vi "SmartInsert.vi"(8 "error in (no error)":errorcluster, 11 "SelList[]":refnum<vi>[](array[refnum])) -> (0 "error out":errorcluster)   [LabVIEW 2014]
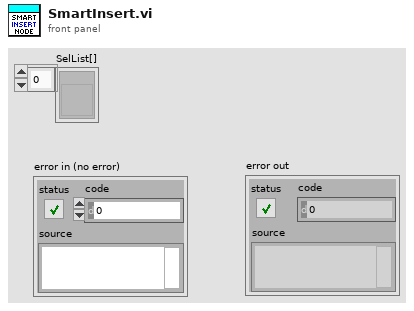
[diagram p1: front panel]
types:
  T1 = cluster{"Source":refnum<vi>, "Sink":refnum<vi>, "Type Variant":variant}
  T2 = cluster{"Position":cluster{"h":i16, "v":i16}, "Flags":i32, "Type":enum32{"LooseEnd", "Endpoint", "Bend", "Junction"}, "Up Joint Index":i16, "Down Joint Index":i16, "Left Joint Index":i16, "Right Joint Index":i16}[]
  T3 = typedef "LVPointTypeDef.ctl" = cluster{"Horizontal":i16, "Vertical":i16}
  T4 = typedef "LVPositionTypeDef.ctl" = cluster{"Left":i32, "Top":i32}
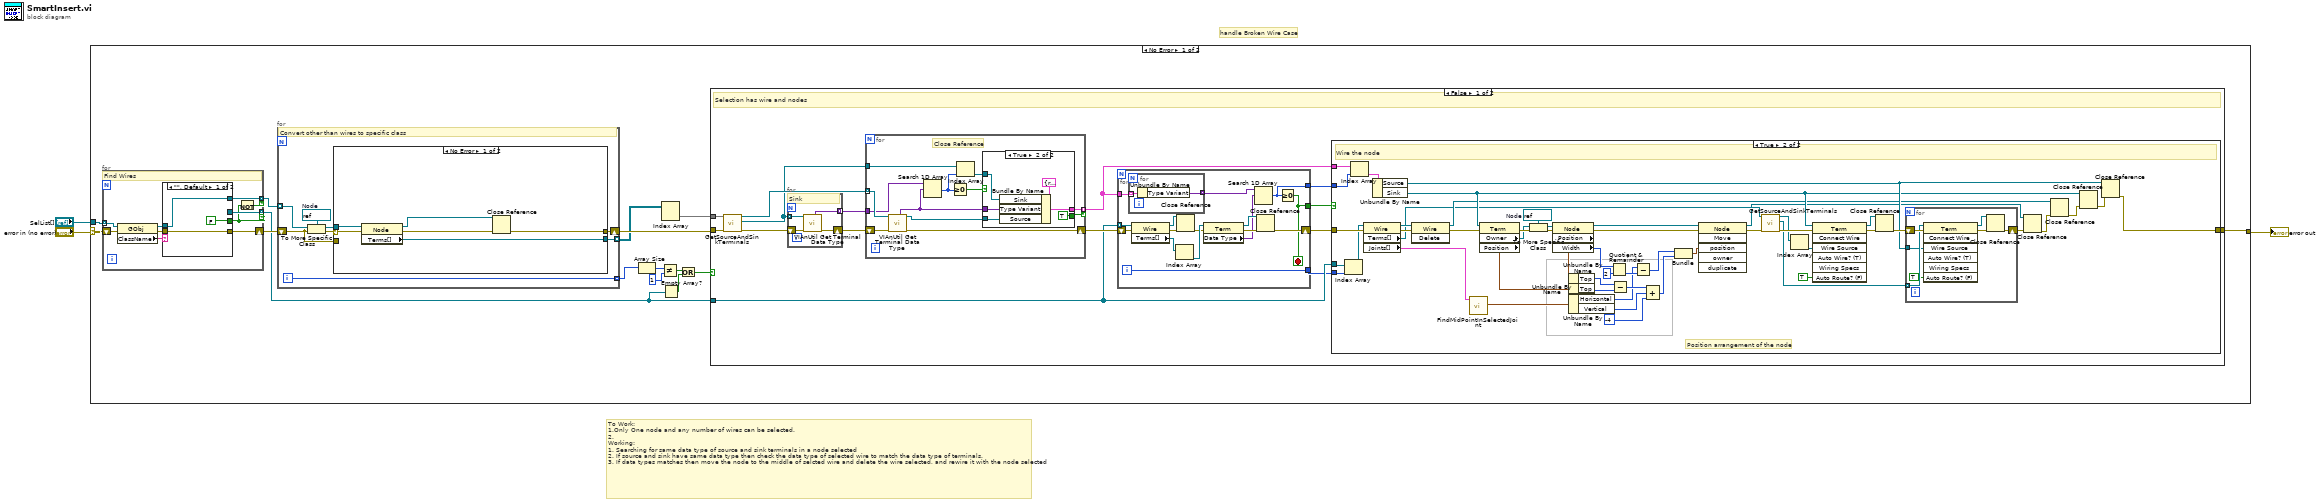
[diagram p0: block diagram]
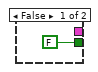
[diagram p3: hidden frame]
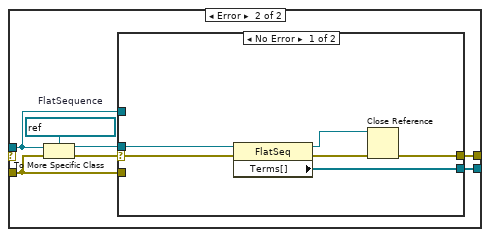
[diagram p5: hidden frame]
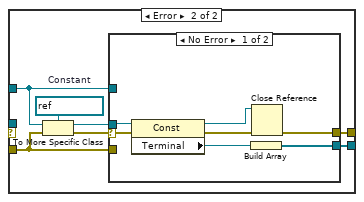
[diagram p6: hidden frame]
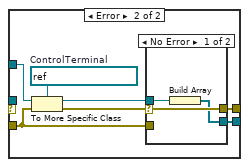
[diagram p7: hidden frame]
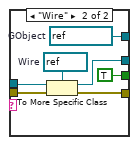
[diagram p9: hidden frame]
diagram:
  # "To Work:\n1.Only One node and any number of wires can be selected.\n2.\nWorking:\n1. Searching for same data type of source and sink terminals in a node selected\n2. If source and sink have same data type then check the data type of selected wire to match the data type of terminals.\n3. If data types matches then move the node to the middle of selcted wire and delete the wire selected, and rewire it with the node selected"
  # "handle Broken Wire Case"
  n1 = case shown="No Error" "error in (no error)" {
    selector: "error in (no error)" -> [w17 w208]
    tunnel: [w10 w208] -> w1
    tunnel: "SelList[]" -> [w18 _]
    frame No Error {
      n2 = for {
        tunnel: w18 -> [w197] mode=indexing
        tunnel: [w191] -> w14 mode=indexing if=w189
        shift-right: [w192] -> w16
        shift-left: w17 -> [w194]
        tunnel: [w190] -> w15 mode=indexing if=w188
        # "Find Wires"
        n3 = property class="GObj"(reference=w197, error in=w194) -> (reference out=w195:refnum<vi>, error out=w193:errorcluster, "ClassName"=w196:string)
        n4 = case shown="\"\", Default" w196 {
          tunnel: w195 -> [w198 w205]
          tunnel: w193 -> [w199 w207]
          tunnel: [w199 w206] -> w192
          tunnel: [_ w203] -> w191
          tunnel: [FALSE TRUE] -> w189
          tunnel: [w198 w201] -> w190
          frame "", Default {
          }
          frame "Wire" {
            w201 = refnum<vi> refnum  # GObject
            w204 = refnum<vi> refnum  # Wire
            n5 = To More Specific Class(target class=w204, reference=w205, error in=w207) -> (specific class reference=w203:refnum<vi>, error out=w206:errorcluster)
          }
        }
        n6 = Not(x=w189) -> (.not. x?=w188:bool)
      }
      n7 = for {
        tunnel: [w141] -> w9 mode=indexing
        shift-right: [w138] -> w11
        shift-left: w16 -> [w139]
        tunnel: w15 -> [w137] mode=indexing
        tunnel: [w136] -> w6 mode=indexing
        i -> [w136]
        w140 = refnum<vi> refnum  # Node
        # "Convert other than wires to specific class"
        n8 = To More Specific Class(target class=w140, reference=w137, error in=w139) -> (specific class reference=w142:refnum<vi>, error out=w143:errorcluster)
        n9 = case shown="No Error" w143 {
          selector: w143 -> [w149 _]
          tunnel: w142 -> [w148 w150]
          tunnel: [w147 w152] -> w141
          tunnel: [w145 w154] -> w138
          tunnel: w139 -> [_ w153]
          frame No Error {
            n10 = property class="Node"(reference=w148, error in=w149) -> (reference out=w144:refnum<vi>, error out=w146:errorcluster, "Terms[]"=w147:refnum<vi>[])
            n11 = Close Reference(reference=w144, error in (no error)=w146) -> (error out=w145:errorcluster)
          }
          frame Error {
            w151 = refnum<vi> refnum  # FlatSequence
            n12 = To More Specific Class(target class=w151, reference=w150, error in=w153) -> (specific class reference=w155:refnum<vi>, error out=w156:errorcluster)
            n13 = case shown="No Error" w156 {
              selector: w156 -> [w162 _]
              tunnel: w155 -> [w161 _]
              tunnel: [w158 w164] -> w154
              tunnel: w153 -> [_ w166]
              tunnel: [w159 w165] -> w152
              tunnel: w150 -> [_ w167]
              frame No Error {
                n14 = property class="FlatSeq"(reference=w161, error in=w162) -> (reference out=w157:refnum<vi>, error out=w160:errorcluster, "Terms[]"=w159:refnum<vi>[])
                n15 = Close Reference(reference=w157, error in (no error)=w160) -> (error out=w158:errorcluster)
              }
              frame Error {
                w163 = refnum<vi> refnum  # Constant
                n16 = To More Specific Class(target class=w163, reference=w167, error in=w166) -> (specific class reference=w168:refnum<vi>, error out=w169:errorcluster)
                n17 = case shown="No Error" w169 {
                  selector: w169 -> [w175 _]
                  tunnel: w168 -> [w176 _]
                  tunnel: w167 -> [_ w183]
                  tunnel: w166 -> [_ w180]
                  tunnel: [w173 w178] -> w165
                  tunnel: [w171 w179] -> w164
                  frame No Error {
                    n18 = property class="Const"(reference=w176, error in=w175) -> (reference out=w170:refnum<vi>, error out=w172:errorcluster, "Terminal"=w174:refnum<vi>)
                    n19 = Build Array(w174) -> (w173:refnum<vi>[])
                    n20 = Close Reference(reference=w170, error in (no error)=w172) -> (error out=w171:errorcluster)
                  }
                  frame Error {
                    w177 = refnum<vi> refnum  # ControlTerminal
                    n21 = To More Specific Class(target class=w177, reference=w183, error in=w180) -> (specific class reference=w181:refnum<vi>, error out=w182:errorcluster)
                    n22 = case shown="No Error" w182 {
                      selector: w182 -> [w186 _]
                      tunnel: w181 -> [w185 _]
                      tunnel: w180 -> [_ w187]
                      tunnel: [w186 w187] -> w179
                      tunnel: [w184 _] -> w178
                      frame No Error {
                        n23 = Build Array(w185) -> (w184:refnum<vi>[])
                      }
                      frame Error {
                      }
                    }
                  }
                }
              }
            }
          }
        }
      }
      n24 = Array Size(array=w6) -> (size(s)=w8:i32)
      n25 = Not Equal?(x=w8, y=1) -> (x != y?=w4:bool)
      n26 = Index Array(array=w9) -> (element=w7:refnum<vi>[])  [unwired: 2 in]
      n27 = Empty Array?(array=w14) -> (empty?=w12:bool)
      n28 = Or(x=w4, y=w12) -> (x .or. y?=w13:bool)
      n29 = case shown="False" w13 {
        tunnel: w14 -> [w24 _]
        tunnel: [w27 w135] -> w10
        tunnel: w11 -> [w33 w135]
        tunnel: w7 -> [w19 _]
        frame False {
          # "Selection has wire and nodes"
          n30 = call "GetSourceAndSinkTerminals.vi"("error in (no error)"=w33, "Terms[]"=w19) -> ("error out"=w31:errorcluster, "Sink"=w20:refnum<vi>[], "Source"=w29:refnum<vi>[])  [unwired: 7 in]
          n31 = for {
            tunnel: w20 -> [w115] mode=indexing
            tunnel: [w114] -> w32 mode=indexing
            shift-right: [w112] -> w30
            shift-left: w31 -> [w113]
            # "Sink"
            n32 = call <vilib>:"VIAnUtil Get Terminal Data Type.vi"("error in (no error)"=w113, "Terminal"=w115) -> ("error out"=w112:errorcluster, "Type Variant"=w114:variant)  [unwired: 6 in, 2 out]
          }
          n33 = for {
            tunnel: w32 -> [w126]
            tunnel: w29 -> [w127] mode=indexing
            shift-right: [w123] -> w28
            shift-left: w30 -> [w124]
            tunnel: w20 -> [w120]
            tunnel: [w117] -> w22 mode=indexing if=w116
            # "Close Reference"
            n34 = call <vilib>:"VIAnUtil Get Terminal Data Type.vi"("error in (no error)"=w124, "Terminal"=w127) -> ("error out"=w123:errorcluster, "dup  Terminal"=w122:refnum<vi>, "Type Variant"=w125:variant)  [unwired: 6 in, 1 out]
            n35 = Search 1D Array(1D array=w126, element=w125) -> (index of element=w121:i32)  [unwired: 1 in]
            n36 = Greater Or Equal To 0?(x=w121) -> (x >= 0?=w118:bool)
            n37 = Index Array(array=w120, index=w121) -> (element=w119:refnum<vi>)
            n38 = case shown="True" w118 {
              tunnel: w125 -> [_ w133]
              tunnel: w122 -> [_ w132]
              tunnel: w119 -> [_ w131]
              tunnel: [_ w130] -> w117
              tunnel: [FALSE TRUE] -> w116
              frame False {
              }
              frame True {
                n39 = Bundle By Name(cluster=T1 {"Source"=refnum, "Sink"=refnum, "Type Variant"=variant}, "Sink"=w131, "Type Variant"=w133, "Source"=w132) -> (w130:T1)
              }
            }
          }
          n40 = for {
            tunnel: w24 -> [w107] mode=indexing
            shift-right: [w103] -> w26
            shift-left: w28 -> [w109]
            tunnel: w22 -> [w101]
            tunnel: [w98] -> w21
            tunnel: [w97] -> w23
            tunnel: [w96] -> w25
            i -> [w97]
            stop <- w96 stop-if-true
            n41 = for {
              tunnel: w101 -> [w111] mode=indexing
              tunnel: [w110] -> w100 mode=indexing
              n42 = Unbundle By Name(w111) -> ("Type Variant"=w110:variant)
            }
            n43 = property class="Wire"(reference=w107, error in=w109) -> (reference out=w94:refnum<vi>, error out=w108:errorcluster, "Terms[]"=w106:refnum<vi>[])
            n44 = Index Array(array=w106) -> (element=w104:refnum<vi>)  [unwired: 1 in]
            n45 = Close Reference(reference=w94, error in (no error)=w108) -> (error out=w95:errorcluster)
            n46 = property class="Term"(reference=w104, error in=w95) -> (reference out=w102:refnum<vi>, error out=w105:errorcluster, "Data Type"=w99:variant)
            n47 = Search 1D Array(1D array=w100, element=w99) -> (index of element=w98:i32)  [unwired: 1 in]
            n48 = Close Reference(reference=w102, error in (no error)=w105) -> (error out=w103:errorcluster)
            n49 = Greater Or Equal To 0?(x=w98) -> (x >= 0?=w96:bool)
          }
          n50 = case shown="True" w25 {
            tunnel: [w34 w71] -> w27
            tunnel: w26 -> [w34 w86]
            tunnel: w24 -> [_ w85]
            tunnel: w23 -> [_ w84]
            tunnel: w22 -> [_ w82]
            tunnel: w21 -> [_ w81]
            frame False {
              # "Discard - Data Type No Matching"
            }
            frame True {
              w63 = refnum<vi> refnum  # Node
              # "Position arrangement of the node"
              # "Wire the node"
              n51 = Index Array(array=w85, index=w84) -> (element=w83:refnum<vi>)
              n52 = Index Array(array=w82, index=w81) -> (element=w80:T1)
              n53 = property class="Wire"(reference=w83, error in=w86) -> (reference out=w67:refnum<vi>, error out=w79:errorcluster, "Terms[]"=w43:refnum<vi>[], "Joints[]"=w66:T2)
              n54 = Unbundle By Name(w80) -> ("Source"=w65:refnum<vi>, "Sink"=w45:refnum<vi>)
              n55 = invoke class="Wire" method="Delete"(reference=w67, error in=w79) -> (reference out=w44:refnum<vi>, error out=w47:errorcluster)  [unwired: 1 in, 1 out]
              n56 = call "FindMidPointInSelectedJoint.vi"("Joints[]"=w66) -> ("MidPoint"=w40:T3)  [unwired: 8 in, 2 out]
              n57 = property class="Term"(reference=w45, error in=w47) -> (error out=w62:errorcluster, "Owner"=w61:refnum<vi>, "Position"=w59:T4)  [unwired: 1 out]
              n58 = To More Specific Class(target class=w63, reference=w61, error in=w62) -> (specific class reference=w52:refnum<vi>, error out=w51:errorcluster)
              n59 = property class="Node"(reference=w52, error in=w51) -> (reference out=w50:refnum<vi>, error out=w49:errorcluster, "Position"=w60:T4, "Width"=w54:u32)
              n60 = Unbundle By Name(w60) -> ("Top"=w58:i32)
              n61 = Unbundle By Name(w59) -> ("Top"=w57:i32)
              n62 = Unbundle By Name(w40) -> ("Horizontal"=w39:i16, "Vertical"=w38:i16)
              n63 = Quotient & Remainder(x=w54, y=u32 2) -> (floor(x/y)=w55:u32)  [unwired: 1 out]
              n64 = Subtract(x=w58, y=w57) -> (x-y=w56:i32)
              n65 = Subtract(x=w39, y=w55) -> (x-y=w37:u32)
              n66 = Compound Arithmetic op=ADD(w56, w38, i16 -4 ("value")) -> (w36:i32)
              n67 = Bundle(w37, w36) -> (w35:cluster{u32, i32})  [unwired: 1 in]
              n68 = invoke class="Node" method="Move"(reference=w50, error in=w49, "position"=w35) -> (reference out=w41:refnum<vi>, error out=w46:errorcluster)  [unwired: 3 in, 4 out]
              n69 = call "GetSourceAndSinkTerminals.vi"("error in (no error)"=w46, "Terms[]"=w43) -> ("error out"=w78:errorcluster, "Sink"=w74:refnum<vi>[], "Source"=w77:refnum<vi>[])  [unwired: 7 in]
              n70 = Index Array(array=w77) -> (element=w76:refnum<vi>)  [unwired: 1 in]
              n71 = invoke class="Term" method="Connect Wire"(reference=w45, error in=w78, "Wire Source"=w76, "Auto Route? (F)"=TRUE) -> (reference out=w69:refnum<vi>, error out=w75:errorcluster)  [unwired: 3 in, 5 out]
              n72 = Close Reference(reference=w69, error in (no error)=w75) -> (error out=w70:errorcluster)
              n73 = for {
                shift-right: [w89] -> w42
                shift-left: w70 -> [w93]
                tunnel: w74 -> [w91] mode=indexing
                tunnel: w65 -> [w90]
                n74 = invoke class="Term" method="Connect Wire"(reference=w91, error in=w93, "Wire Source"=w90, "Auto Route? (F)"=TRUE) -> (reference out=w88:refnum<vi>, error out=w92:errorcluster)  [unwired: 3 in, 5 out]
                n75 = Close Reference(reference=w88, error in (no error)=w92) -> (error out=w89:errorcluster)
              }
              n76 = Close Reference(reference=w41, error in (no error)=w42) -> (error out=w64:errorcluster)
              n77 = Close Reference(reference=w44, error in (no error)=w64) -> (error out=w73:errorcluster)
              n78 = Close Reference(reference=w45, error in (no error)=w73) -> (error out=w72:errorcluster)
              n79 = Close Reference(reference=w65, error in (no error)=w72) -> (error out=w71:errorcluster)
            }
          }
        }
        frame True {
          # "No Nodes or Wires in selection. Discard"
        }
      }
    }
    frame Error {
    }
  }
  "error out" <- w1
